vi "DVR Unflatten.vi"(7 "Header in":T1, 8 "error in (no error)":errorcluster, 10 "DVRs In":refnum<data-value>[](array[refnum]), 11 "Flatten Data in":u8[](array[numeric])) -> (0 "error out":errorcluster, 2 "DVRs Out":refnum<data-value>[](array[refnum]), 3 "Flatten Data out":u8[](array[numeric]), 5 "Header out":T1)   [LabVIEW 2021, in "CIFfifo.lvclass"]
uses:
  CIFfifo.lvclass
  typedef/FIFO Header.ctl
  typedef/Datatype Waveform.ctl
  CIFCore/Common/Typedef/Errors.ctl
  <vilib>/CIF Foundation/CIF Utilities/Errors/Append Error Location.vi
  ChannelCommon.lvlib
  CIFCore/Common/CIFCoreCommon.lvlib
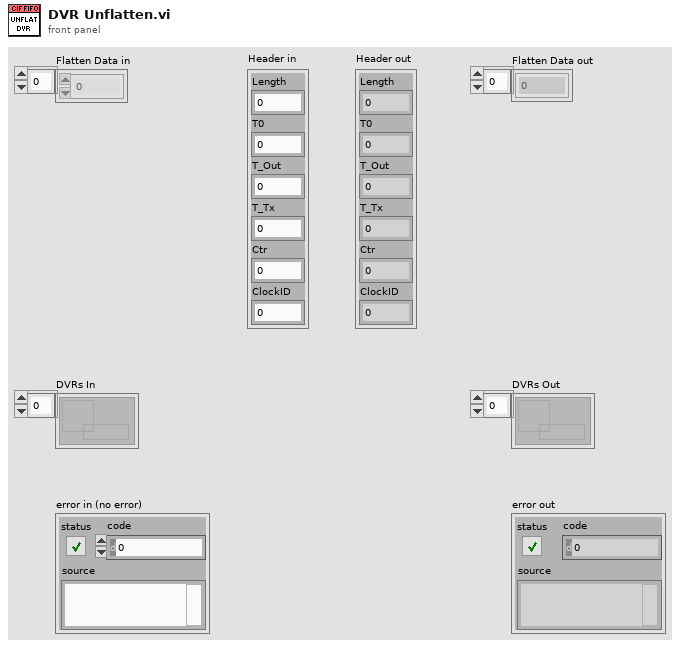
[diagram p1: front panel]
types:
  T1 = typedef "ChannelCommon.lvlib/FIFO Header.ctl" = cluster{"Length":u64, "T0":i64, "T_Out":i64, "T_Tx":i64, "Ctr":u64, "ClockID":u8}
  T2 = typedef "CIFCoreCommon.lvlib/Errors.ctl" = enum16{"Invalid Clock ID", "Long Sleep", "gRPC Server Not Found", "Config Parse", "Timestamp Wrap", "Delayed Execution", "Duplicate Channel", "Missing Channel", "Incorrect Type", "Flatten Error", "Unflatten Data", "Unique Name", "Plugin Not Found", "Plugin Type Not Found", "Plugin Version Not Found", "Manager Not Found", "Numerical Issue", "Time Jump", "Clock ID Match", "Channel Length", "Plugin Connection", "gRPC Server Connection", "PPL Name Match", "Build", "Config Log Parse"}
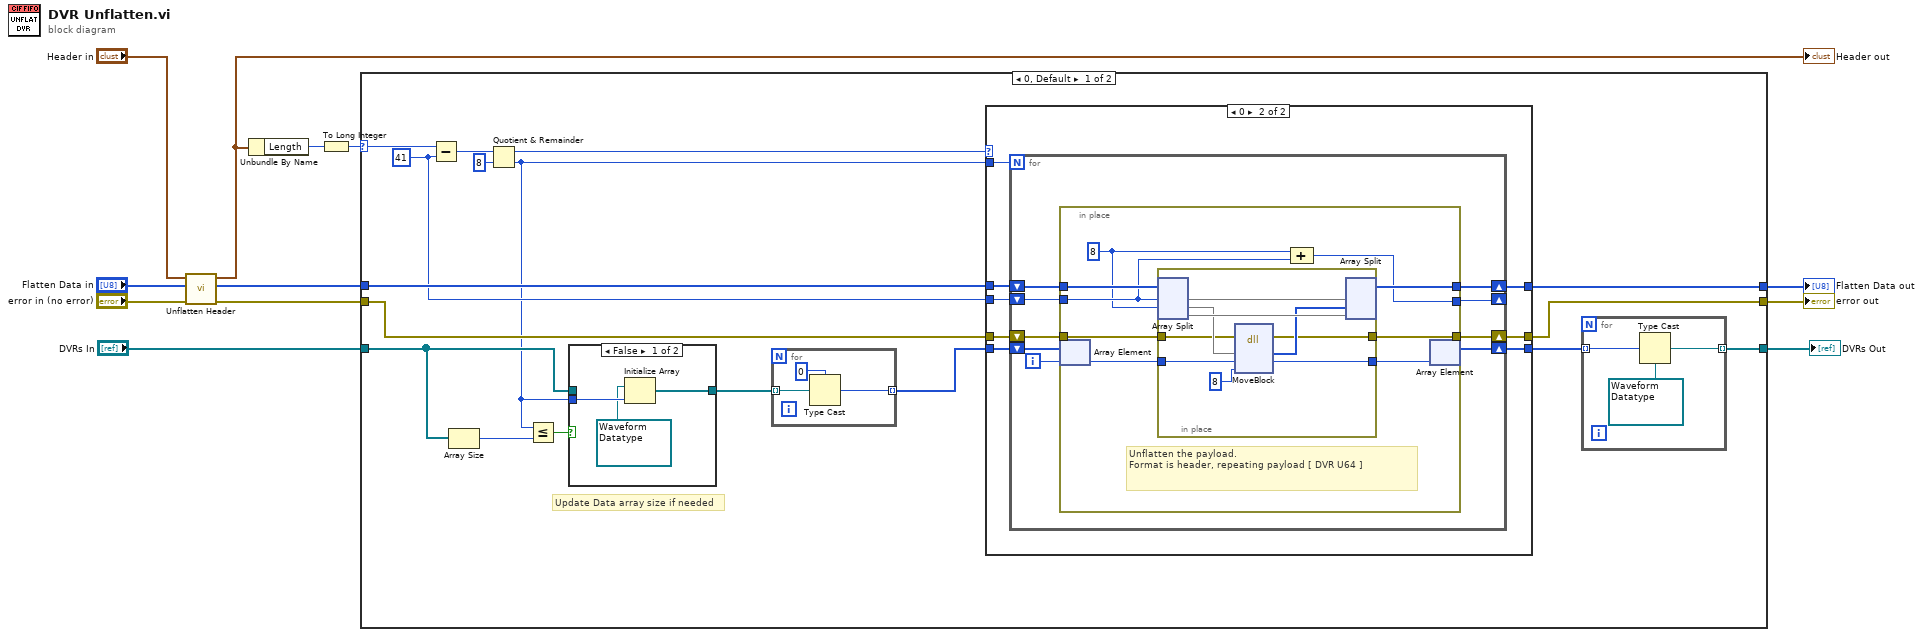
[diagram p0: block diagram]
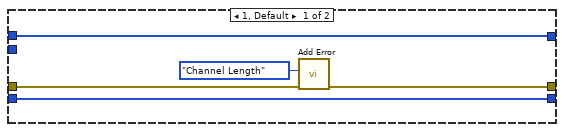
[diagram p2: hidden frame]
diagram:
  n1 = call "Unflatten Header.vi"("error in"="error in (no error)", "Flattened Data in"="Flatten Data in", "Header in"="Header in") -> ("error out"=w8:errorcluster, "Flatten Data out"=w10:u8[], "Header out"=w5:T1)  [unwired: 6 in]
  "Header out" <- w5
  n2 = Unbundle By Name(w5) -> ("Length"=w6:u64)
  n3 = To Long Integer(number=w6) -> (32bit integer=w4:i32)
  n4 = case shown="0, Default" w4 {
    selector: w4 -> [w25 _]
    tunnel: [w13 w80] -> w1
    tunnel: "DVRs In" -> [w19 w80]
    tunnel: [w29 w81] -> w12
    tunnel: [w28 w82] -> w11
    tunnel: w10 -> [w27 w82]
    tunnel: w8 -> [w26 w81]
    frame 0, Default {
      w24 = 41
      # "Update Data array size if needed"
      n5 = Subtract(x=w25, y=w24) -> (x-y=w23:i32)
      n6 = Array Size(array=w19) -> (size(s)=w21:i32)
      n7 = Quotient & Remainder(x=w23, y=8) -> (x-y*floor(x/y)=w17:i32, floor(x/y)=w18:i32)
      n8 = Less Or Equal?(x=w18, y=w21) -> (x <= y?=w20:bool)
      n9 = case shown="False" w20 {
        tunnel: w19 -> [_ w79]
        tunnel: [w78 w79] -> w16
        tunnel: w18 -> [w77 _]
        frame False {
          n10 = Initialize Array(refnum<data-value> refnum ("element"), w77) -> (w78:refnum<data-value>[])
        }
        frame True {
        }
      }
      n11 = for {
        tunnel: w16 -> [w35] mode=indexing
        tunnel: [w33] -> w15 mode=indexing
        n12 = Type Cast(type=u64 0, x=w35) -> (*(type *) &x=w33:u64)
      }
      n13 = case shown="0" w17 {
        tunnel: [w38 w48] -> w14
        tunnel: [w37 w47] -> w29
        tunnel: [w40 w46] -> w28
        tunnel: w27 -> [w40 w45]
        tunnel: w26 -> [w39 w44]
        tunnel: w24 -> [_ w43]
        tunnel: w15 -> [w38 w42]
        tunnel: w18 -> [_ w41]
        frame 1, Default {
          n14 = call "Add Error.vi"("error in (no error)"=w39, "Error"=Errors."Channel Length") -> ("error out"=w37:errorcluster)  [unwired: 9 in]
        }
        frame 0 {
          n15 = for {
            N: w41 -> [_]
            shift-right: [w49] -> w47
            shift-left: w44 -> [w54]
            shift-right: [w57] -> w46
            shift-left: w45 -> [w56]
            shift-right: [w53] -> _
            shift-left: w43 -> [w55]
            shift-right: [w50] -> w48
            shift-left: w42 -> [w51]
            i -> [w52]
            n16 = in-place {
              in-place-border: [w66] -> w57
              in-place-border: w56 -> [w65]
              in-place-border: w55 -> [w64]
              in-place-border: w54 -> [w63]
              in-place-border: [w62] -> w53
              in-place-border: [w58] -> w49
              w61 = 8 ("y")
              # "Unflatten the payload.\nFormat is header, repeating payload [ DVR U64 ]"
              n17 = in-place-array #1(w51, w52) -> (w60:u64)
              n18 = in-place {
                in-place-border: [w74] -> w59
                in-place-border: w63 -> [w68]
                in-place-border: w60 -> [w69]
                in-place-border: [w67] -> w58
                n19 = in-place-split #2(w65, w64, w61) -> (w75:u8[], w71:u8[], w72:u8[])
                n20 = dll-call lib="LabVIEW" fn="MoveBlock"(error in=w68, "source"=w71, "dest"=w69, "size"=u64 8) -> (error out=w67:errorcluster, "source"=w70:u8[], "dest"=w74:u64)  [unwired: 4 in, 1 out]
                n21 = in-place-split #2(w75, w70, w72) -> (w66:u8[])  [unwired: 2 out]
              }
              n22 = Compound Arithmetic op=ADD(w61, w64) -> (w62:i32)
              n23 = in-place-array #1(w59) -> (w50:u64[])  [unwired: 1 out]
            }
          }
        }
      }
      n24 = for {
        tunnel: w14 -> [w32] mode=indexing
        tunnel: [w31] -> w13 mode=indexing
        n25 = Type Cast(type=refnum<data-value> refnum ("element"), x=w32) -> (*(type *) &x=w31:refnum<data-value>)
      }
    }
    frame 40 {
      # "Header only"
    }
  }
  "error out" <- w12
  "Flatten Data out" <- w11
  "DVRs Out" <- w1
